vi "Get Owner.vi"(8 "error in (no error)":errorcluster, 11 "ArrayPanel in":refnum<class "ArrayPanel.lvclass">) -> (0 "error out":errorcluster, 2 "Owner":refnum<class>, 3 "ArrayPanel out":refnum<class "ArrayPanel.lvclass">)   [LabVIEW 2020, in "OOPanel.lvlib" / "ArrayPanel.lvclass"]
uses:
  ArrayPanel.lvclass
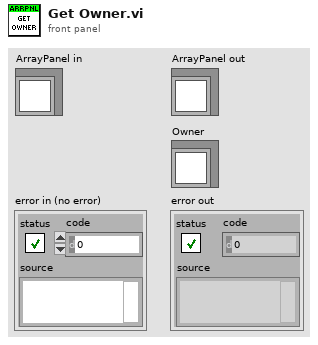
[diagram p1: front panel]
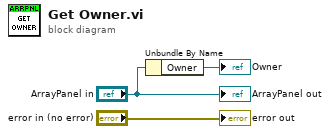
[diagram p0: block diagram]
diagram:
  n1 = Unbundle By Name("ArrayPanel in") -> ("Owner"=→"Owner":refnum<class>)
  "error out" <- "error in (no error)"
  "ArrayPanel out" <- "ArrayPanel in"
